vi "ROI entry-Get ROI indices.vi"(6 "Z stop code":u8, 7 "Z start code":u8, 10 "Z stop index":i32, 11 "Z start Index":i32) -> (2 "Z codes":u8[](array[numeric]), 3 "Z Idx(s)":i32[](array[numeric]))   [LabVIEW 2020]
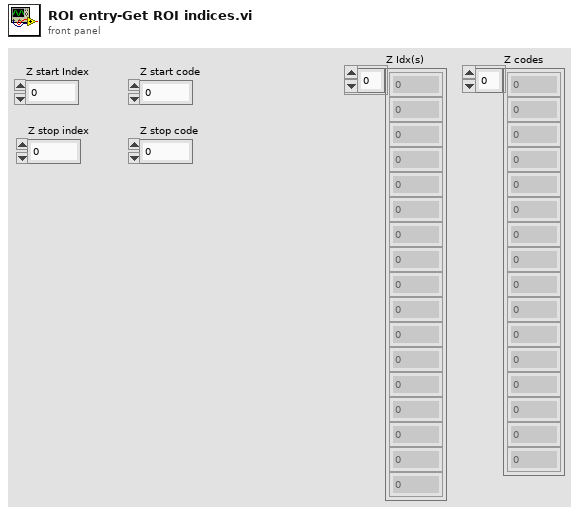
[diagram p1: front panel]
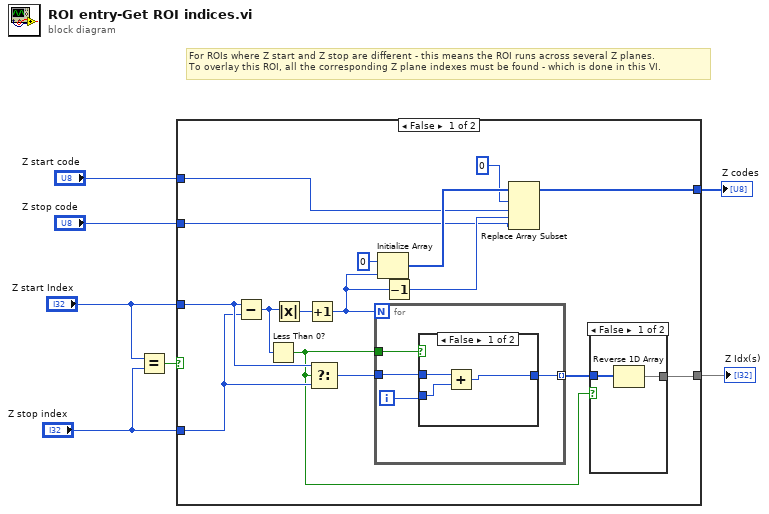
[diagram p0: block diagram]
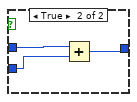
[diagram p3: hidden frame]
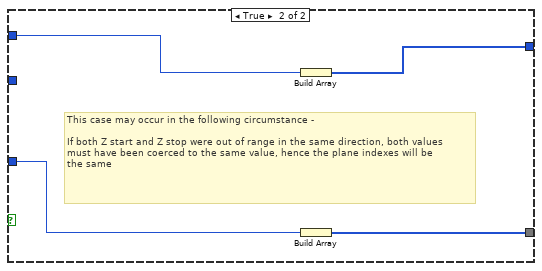
[diagram p4: hidden frame]
diagram:
  # "For ROIs where Z start and Z stop are different - this means the ROI runs across several Z planes.\nTo overlay this ROI, all the corresponding Z plane indexes must be found - which is done in this VI."
  n1 = Equal?(x="Z start Index", y="Z stop index") -> (x = y?=w6:bool)
  n2 = case shown="False" w6 {
    tunnel: "Z start Index" -> [w21 w40]
    tunnel: "Z stop index" -> [w20 _]
    tunnel: [w10 w39] -> w7
    tunnel: "Z start code" -> [w9 w38]
    tunnel: [w13 w37] -> w2
    tunnel: "Z stop code" -> [w8 _]
    frame False {
      n3 = Subtract(x=w21, y=w20) -> (x-y=w23:i32)
      n4 = Less Than 0?(x=w23) -> (x < 0?=w12:bool)
      n5 = Absolute Value(x=w23) -> (abs(x)=w19:i32)
      n6 = Increment(x=w19) -> (x+1=w15:i32)
      n7 = Select(t=w21, s=w12, f=w20) -> (s? t:f=w22:i32)
      n8 = for {
        N: w15 -> [_]
        tunnel: w22 -> [w30]
        tunnel: [w29] -> w11 mode=indexing
        tunnel: w12 -> [w28]
        i -> [w27]
        n9 = case shown="False" w28 {
          tunnel: w30 -> [w33 w36]
          tunnel: [w32 w34] -> w29
          tunnel: w27 -> [w31 w35]
          frame False {
            n10 = Add(x=w33, y=w31) -> (x+y=w32:i32)
          }
          frame True {
            n11 = Add(x=w36, y=w35) -> (x+y=w34:i32)
          }
        }
      }
      n12 = Initialize Array(u8 0 ("element"), w15) -> (w17:u8[])
      n13 = Decrement(x=w15) -> (x-1=w14:i32)
      n14 = Replace Array Subset(array=w17, new element #1=w9, index #1=0 ("index"), new element #2=w8, index #2=w14) -> (w13:u8[])
      n15 = case shown="False" w12 {
        tunnel: w11 -> [w25 w26]
        tunnel: [w24 w26] -> w10
        frame False {
          n16 = Reverse 1D Array(array=w25) -> (reversed array=w24:i32[])
        }
        frame True {
        }
      }
    }
    frame True {
      # "This case may occur in the following circumstance - \n\nIf both Z start and Z stop were out of range in the same direction, both values\nmust have been coerced to the same value, hence the plane indexes will be \nthe same"
      n17 = Build Array(w38) -> (w37:u8[])
      n18 = Build Array(w40) -> (w39:i32[])
    }
  }
  "Z Idx(s)" <- w7
  "Z codes" <- w2
